vi "Pre-Process.vi"(11 "TEMPLATE Actor in":refnum<class "TEMPLATE Actor.lvclass">) -> (3 "TEMPLATE Actor out":refnum<class "TEMPLATE Actor.lvclass">)   [LabVIEW 2020, in "_Template.lvlib" / "Templates.lvlib" / "TEMPLATE Actor.lvlib" / "TEMPLATE Actor.lvclass"]
uses:
  TEMPLATE Actor.lvclass
  jettl/jettl/Actor/Actor/Actor.lvclass
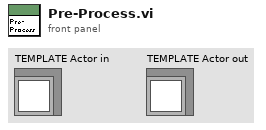
[diagram p1: front panel]
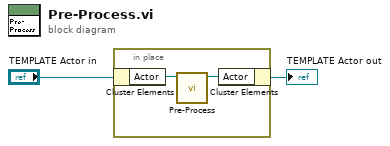
[diagram p0: block diagram]
diagram:
  n1 = in-place {
    n2 = in-place-cluster #1("TEMPLATE Actor in") -> ("Actor"=w4:refnum<class "Actor.lvclass">)
    n3 = call-dynamic "Pre-Process.vi"("Actor in"=w4) -> ("Actor out"=w3:refnum<class "Actor.lvclass">)  [unwired: 10 in]
    n4 = in-place-cluster #1("Actor"=w3) -> (→"TEMPLATE Actor out":refnum<class "TEMPLATE Actor.lvclass">)
  }
